vi "Write Hardware part number.vi"(6 "error in":errorcluster, 7 "HW part number":string, 8 "MaxRead":i32, 9 "Channel in":u16) -> (0 "error out":errorcluster, 1 "Messages":T1(array[cluster]), 2 "Pass":bool, 3 "Channel out":u16)   [LabVIEW 2023]
uses:
  4f930f32-d09a-43ef-bca1-8b214b378bd5.vi
  Communication/PCAN2023/PCAN API.lvlib
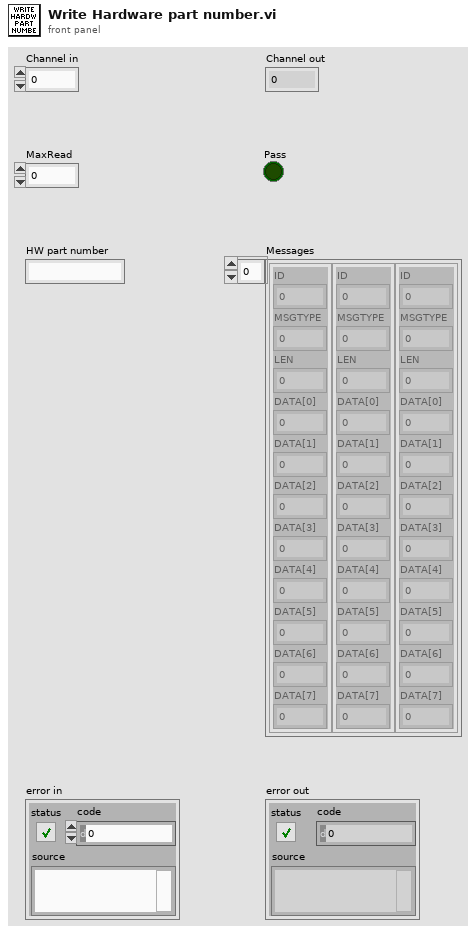
[diagram p1: front panel]
types:
  T1 = cluster{"ID":u32, "MSGTYPE":u8, "LEN":u8, "DATA[0]":u8, "DATA[1]":u8, "DATA[2]":u8, "DATA[3]":u8, "DATA[4]":u8, "DATA[5]":u8, "DATA[6]":u8, "DATA[7]":u8}[]
  T2 = cluster{"ID":u32, "MSGTYPE":u8, "LEN":u8, "DATA[0]":u8, "DATA[1]":u8, "DATA[2]":u8, "DATA[3]":u8, "DATA[4]":u8, "DATA[5]":u8, "DATA[6]":u8, "DATA[7]":u8}
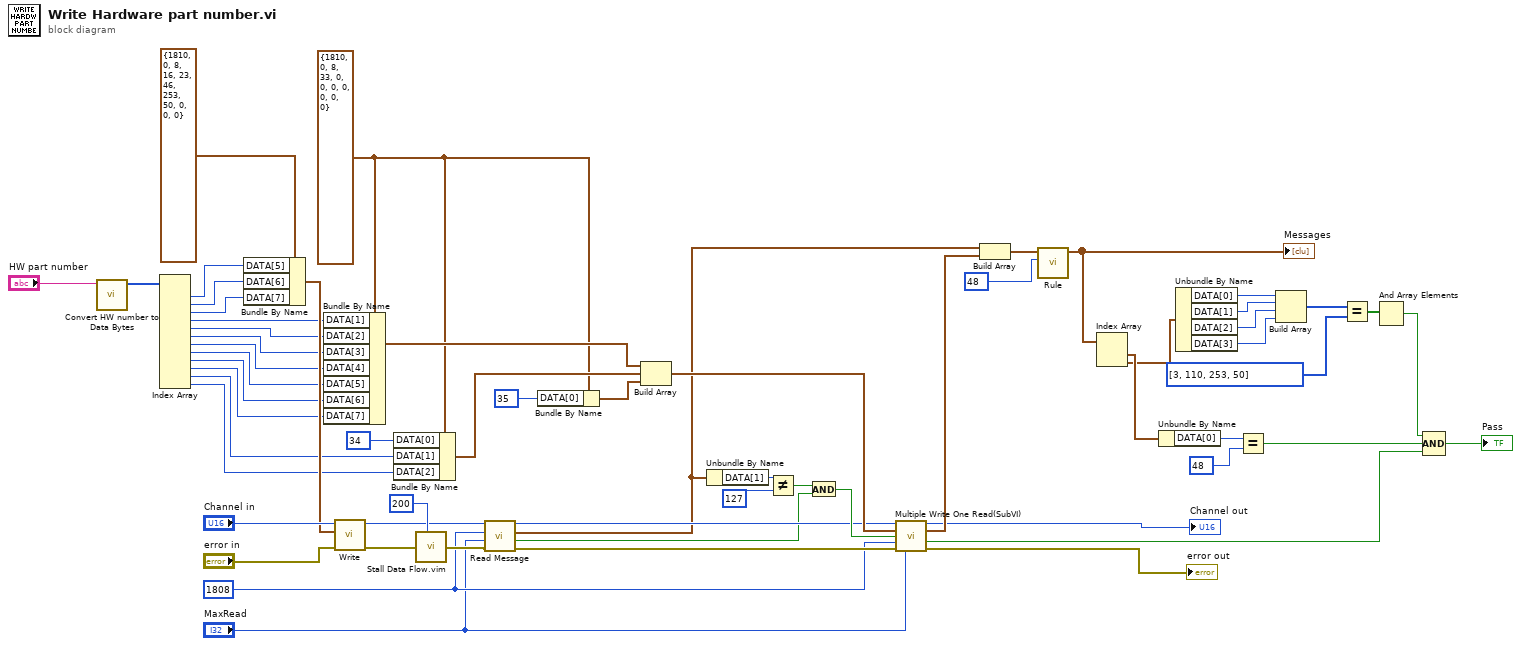
[diagram p0: block diagram]
diagram:
  w21 = T2 {"ID"=1810, "MSGTYPE"=0, "LEN"=8, "DATA[0]"=33, "DATA[1]"=0, "DATA[2]"=0, "DATA[3]"=0, "DATA[4]"=0, "DATA[5]"=0, "DATA[6]"=0, "DATA[7]"=0} ("MessageBuffer")
  (unwired) u32 200 ("milliseconds to wait")
  w7 = u32 1808 ("ID")
  n1 = call "Convert HW number to Data Bytes.vi"("HW part number"="HW part number") -> ("ASCII"=w34:u8[])  [unwired: 10 in]
  n2 = Index Array(array=w34) -> (element #1=w37:u8, element #2=w36:u8, element #3=w35:u8, element #4=w32:u8, element #5=w31:u8, element #6=w30:u8, element #7=w29:u8, element #8=w28:u8, element #9=w27:u8, element #10=w26:u8, element #11=w24:u8, element #12=w23:u8)  [unwired: 12 in]
  n3 = Bundle By Name(cluster=T2 {"ID"=1810, "MSGTYPE"=0, "LEN"=8, "DATA[0]"=16, "DATA[1]"=23, "DATA[2]"=46, "DATA[3]"=253, "DATA[4]"=50, "DATA[5]"=0, "DATA[6]"=0, "DATA[7]"=0} ("MessageBuffer"), "DATA[5]"=w37, "DATA[6]"=w36, "DATA[7]"=w35) -> (w52:T2)
  n4 = Bundle By Name(cluster=w21, "DATA[1]"=w32, "DATA[2]"=w31, "DATA[3]"=w30, "DATA[4]"=w29, "DATA[5]"=w28, "DATA[6]"=w27, "DATA[7]"=w26) -> (w33:T2)
  n5 = call "Write.vi"("error in"="error in", "MessageBuffer"=w52, "Channel"="Channel in") -> ("error out"=w56:errorcluster, "Channel out"=w13:u16)  [unwired: 5 in, 2 out]
  n6 = Bundle By Name(cluster=w21, "DATA[0]"=u8 34, "DATA[1]"=w24, "DATA[2]"=w23) -> (w22:T2)
  n7 = call "Stall Data Flow.vim"("value in"=w56, "milliseconds to wait"=u32 200) -> ("value out"=w8:errorcluster)  [unwired: 1 out]
  n8 = call "Read Message.vi"("error in"=w8, "MaxRead"="MaxRead", "ID"=w7, "Channel in"=w13) -> ("error out"=w10:errorcluster, "Passed"=w9:bool, "Last Message"=w11:T2, "Channel out"=w12:u16)  [unwired: 3 in, 1 out]
  n9 = Bundle By Name(cluster=w21, "DATA[0]"=u8 35) -> (w50:T2)
  n10 = Build Array(w33, w22, w50) -> (w20:T1)
  n11 = Unbundle By Name(w11) -> ("DATA[1]"=w55:u8)
  n12 = Not Equal?(x=w55, y=u8 127) -> (x != y?=w19:bool)
  n13 = And(x=w19, y=w9) -> (x .and. y?=w18:bool)
  n14 = call "Multiple Write One Read(SubVI).vi"("Channel in"=w12, "Messages to write"=w20, "Mess 1 Passed"=w18, "ID"=w7, "error in"=w10, "MaxRead"="MaxRead") -> ("Channel out"=→"Channel out":u16, "Last Message"=w17:T2, "Messages passed"=w14:bool, "error out"=→"error out":errorcluster)  [unwired: 6 in]
  n15 = Build Array(w11, w17) -> (w5:T1)
  n16 = call "Rule.vi"("Case"=u8 48 ("y"), "Array in"=w5) -> ("Array out"=w4:T1)  [unwired: 9 in]
  "Messages" <- w4
  n17 = Index Array(array=w4) -> (element #1=w3:T2, element #2=w2:T2)  [unwired: 2 in]
  n18 = Unbundle By Name(w3) -> ("DATA[0]"=w47:u8)
  n19 = Unbundle By Name(w2) -> ("DATA[0]"=w46:u8, "DATA[1]"=w45:u8, "DATA[2]"=w44:u8, "DATA[3]"=w43:u8)
  n20 = Equal?(x=w47, y=u8 48) -> (x = y?=w49:bool)
  n21 = Build Array(w46, w45, w44, w43) -> (w42:u8[])
  n22 = Equal?(x=w42, y=u8[] [3, 110, 253, 50]) -> (x = y?=w40:bool[])
  n23 = And Array Elements(Boolean array=w40) -> (logical AND=w39:bool)
  n24 = Compound Arithmetic op=AND(w39, w49, w14) -> (→"Pass":bool)
